vi "Powerstab.vi"(8 "error out":errorcluster, 10 "Power precision":dbl=0.1, 11 "Laser Power [W]":dbl format="%#.2g") -> (0 "error out 2":errorcluster, 3 "Finshed?":bool)   [LabVIEW 2011]
uses:
  monochromatorcontrol/perHandlemonochromator.vi
  GlobalVar.vi
  monochromatorcontrol/libPhyspec.lvlib
panel:
  out "error-1":dbl
  out "sum":dbl
  out "In Range?":bool
  out "Laser Q":dbl
  out "Laser Power":u8(slide) scale=0.0..2350.0
  out "Current Power":dbl
  out "Current Wavelength":dbl
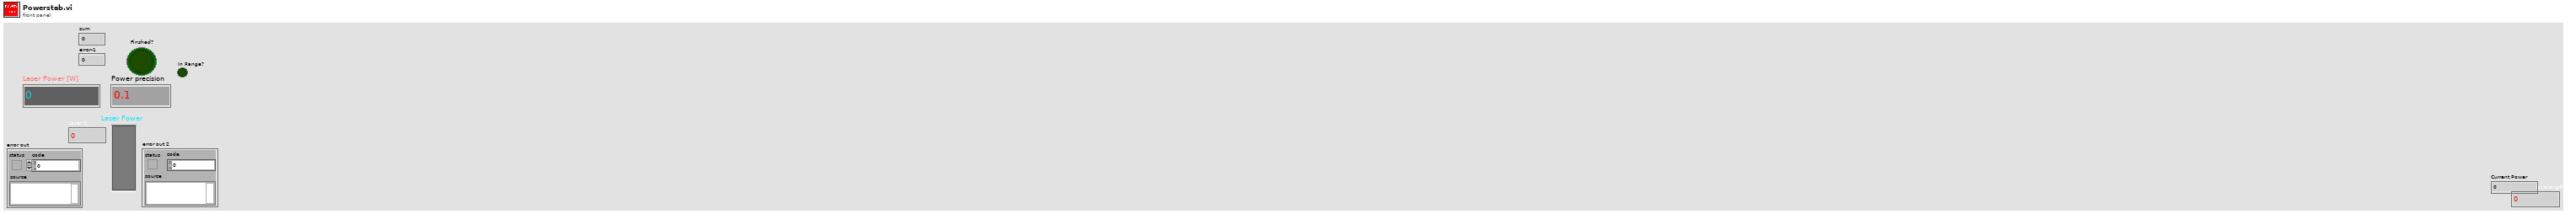
[diagram p1: front panel]
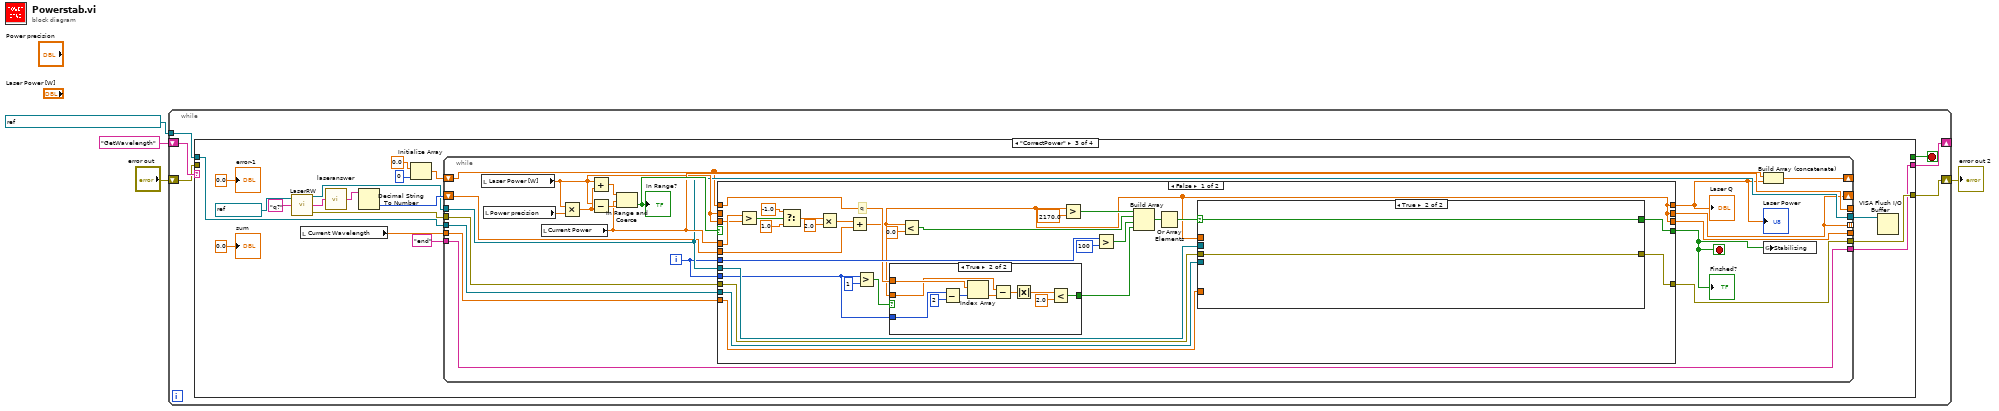
[diagram p0: block diagram]
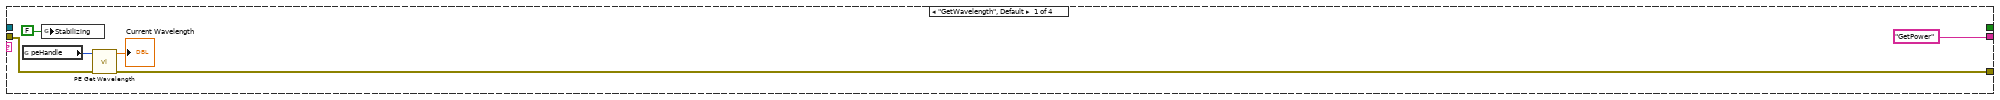
[diagram p2: hidden frame]
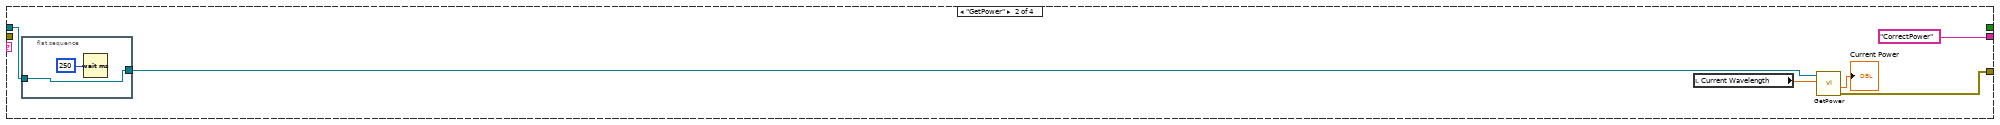
[diagram p3: hidden frame]
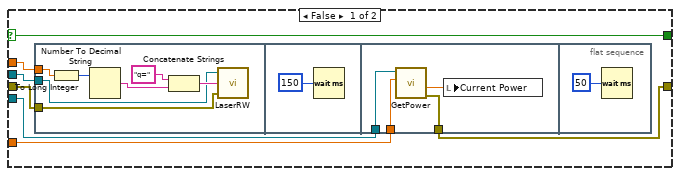
[diagram p5: hidden frame]
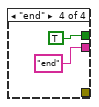
[diagram p7: hidden frame]
diagram:
  n1 = while {
    shift-right: [w7] -> _
    shift-left: "GetWavelength" -> [w10]
    shift-right: [w8] -> w1
    shift-left: "error out" -> [w9]
    tunnel: refnum<visa-resource-name> "USB0::0x1313::0x8072::P2007928::INSTR" ("Input Device") -> [w6]
    stop <- w5 stop-if-true
    n2 = case shown="\"CorrectPower\"" w10 {
      tunnel: w9 -> [w14 _ _ _]
      tunnel: [w13 w18 w27 _] -> w8
      tunnel: ["GetPower" "CorrectPower" w25 "end"] -> w7
      tunnel: w6 -> [_ w20 w29 _]
      tunnel: [_ _ _ TRUE] -> w5
      frame "GetWavelength", Default {
        n3 = global read "perHandlemonochromator.vi" "peHandle"() -> (w16:u32)
        n4 = global write "GlobalVar.vi" "Stabilizing"(FALSE ("Stabilizing")) -> ()
        n5 = call "PE Get Wavelength.vi"("error in (no error)"=w14, "peHandle"=w16) -> ("error out"=w13:errorcluster, "wavelength"=→"Current Wavelength":dbl)  [unwired: 7 in, 1 out]
      }
      frame "GetPower" {
        n6 = flat-sequence {
          tunnel: [w23] -> w21
          tunnel: w20 -> [w23]
          frame #0 {
            n7 = Wait (ms)(milliseconds to wait=u32 250) -> ()  [unwired: 1 out]
          }
        }
        n8 = local read "Current Wavelength"() -> (w19:dbl)
        n9 = call "GetPower.vi"("Wavelength (nm)"=w19, "Input Device"=w21) -> ("error out"=w18:errorcluster, "Power (W)"=→"Current Power":dbl)  [unwired: 2 in, 2 out]
      }
      frame "CorrectPower" {
        n10 = call "LaserRW.vi"("buffer à écrire"="q?", "Nom de ressource VISA"=refnum<visa-resource-name> "COM19") -> ("error out"=w36:errorcluster, "buffer lu"=w38:string, "Nom de ressource VISA en sortie"=w37:refnum<visa-resource-name>)  [unwired: 1 in]
        n11 = local read "Current Wavelength"() -> (w28:dbl)
        n12 = call "laseranswer.vi"("IN"=w38) -> ("Answer"=w35:string)
        n13 = Decimal String To Number(string=w35) -> (number=w39:i32)  [unwired: 2 in, 1 out]
        n14 = Initialize Array(0.0 ("element"), 0 ("dimension size")) -> (w31:dbl[])
        n15 = while {
          tunnel: [w58] -> _
          tunnel: w29 -> [w57]
          tunnel: w28 -> [w56]
          tunnel: [w55] -> _
          tunnel: w37 -> [w53]
          tunnel: [w53] -> w40
          shift-right: [w51] -> _
          shift-left: w39 -> [w50]
          tunnel: w36 -> [w52]
          tunnel: [w51] -> _ mode=indexing
          shift-right: [w48] -> _
          shift-left: w31 -> [w49]
          tunnel: [w45] -> w27
          tunnel: "end" -> [w44]
          tunnel: [w44] -> w25
          i -> [w47]
          stop <- w43 stop-if-true
          n16 = local read "Laser Power [W]"() -> (w54:dbl)
          n17 = local read "Power precision"() -> (w63:dbl)
          n18 = local read "Current Power"() -> (w58:dbl)
          n19 = Multiply(x=w54, y=w63) -> (x*y=w60:dbl)
          n20 = Add(x=w54, y=w60) -> (x+y=w61:dbl)
          n21 = Subtract(x=w54, y=w60) -> (x-y=w62:dbl)
          n22 = In Range and Coerce(upper limit=w61, x=w58, lower limit=w62) -> (In Range?=w59:bool)  [unwired: 1 out]
          "In Range?" <- w59
          n23 = case shown="False" w59 {
            selector: w59 -> [_ w129]
            tunnel: [w87 w129] -> w43
            tunnel: w58 -> [w86 _]
            tunnel: w54 -> [_ _]
            tunnel: w57 -> [w91 _]
            tunnel: w56 -> [w90 _]
            tunnel: w50 -> [w78 w128]
            tunnel: w53 -> [w92 _]
            tunnel: [w65 w128] -> w55
            tunnel: w47 -> [w71 _]
            tunnel: w54 -> [w85 _]
            tunnel: [w65 w128] -> w46
            tunnel: [w65 w128] -> w51
            tunnel: w52 -> [w77 w127]
            tunnel: w49 -> [w70 _]
            tunnel: w47 -> [w67 _]
            tunnel: [w64 w127] -> w45
            frame False {
              # "q"
              n24 = Greater?(x=w86, y=w85) -> (0:w84:bool)
              n25 = Select(t=-1.0, s=w84, f=1.0) -> (s? t:f=w81:dbl)
              n26 = Multiply(x=w81, y=2.0) -> (x*y=w79:dbl)
              n27 = Add(x=w79, y=w78) -> (x+y=w65:dbl)
              n28 = Greater?(x=w67, y=1) -> (0:w68:bool)
              n29 = case shown="True" w68 {
                selector: w68 -> [w94 _]
                tunnel: w70 -> [_ w103]
                tunnel: w67 -> [_ w102]
                tunnel: [w94 w95] -> w66
                tunnel: w65 -> [_ w101]
                frame False {
                }
                frame True {
                  n30 = Subtract(x=w102, y=2) -> (x-y=w104:i32)
                  n31 = Index Array(array=w103, index=w104) -> (element=w100:dbl)
                  n32 = Subtract(x=w101, y=w100) -> (x-y=w99:dbl)
                  n33 = Absolute Value(x=w99) -> (abs(x)=w96:dbl)
                  n34 = Less?(x=w96, y=2.0) -> (x < y?=w95:bool)
                }
              }
              n35 = Less?(x=w65, y=0.0) -> (x < y?=w75:bool)
              n36 = Greater?(x=w65, y=2170.0) -> (0:w76:bool)
              n37 = Greater?(x=w71, y=u32 100) -> (0:w74:bool)
              n38 = Build Array(w76, w75, w74, w66) -> (w73:bool[])
              n39 = Or Array Elements(Boolean array=w73) -> (logical OR=w72:bool)
              n40 = case shown="True" w72 {
                selector: w72 -> [w108 w126]
                tunnel: w92 -> [w111 _]
                tunnel: w91 -> [w110 _]
                tunnel: w90 -> [w109 _]
                tunnel: [w108 w126] -> w87
                tunnel: w77 -> [w107 w125]
                tunnel: w65 -> [w106 _]
                tunnel: [w105 w125] -> w64
                frame False {
                  n41 = flat-sequence {
                    tunnel: w111 -> [w113]
                    tunnel: w107 -> [w112]
                    tunnel: w106 -> [w114]
                    tunnel: w110 -> [w123]
                    tunnel: w109 -> [w122]
                    tunnel: [w120] -> w105
                    frame #0 {
                      n42 = To Long Integer(number=w114) -> (32bit integer=w117:i32)
                      n43 = Number To Decimal String(number=w117) -> (decimal integer string=w116:string)  [unwired: 1 in]
                      n44 = Concatenate Strings("q=" ("buffer à écrire"), w116) -> (w115:string)
                      n45 = call "LaserRW.vi"("error in (no error)"=w112, "buffer à écrire"=w115, "Nom de ressource VISA"=w113) -> ()  [unwired: 3 out]
                    }
                    frame #1 {
                      n46 = Wait (ms)(milliseconds to wait=u32 150) -> ()  [unwired: 1 out]
                    }
                    frame #2 {
                      n47 = call "GetPower.vi"("Wavelength (nm)"=w122, "Input Device"=w123) -> ("error out"=w120:errorcluster, "Power (W)"=w121:dbl)  [unwired: 2 in, 2 out]
                      n48 = local write "Current Power"(w121) -> ()
                    }
                    frame #3 {
                      n49 = Wait (ms)(milliseconds to wait=u32 50) -> ()  [unwired: 1 out]
                    }
                  }
                }
                frame True {
                }
              }
            }
            frame True {
            }
          }
          "Laser Q" <- w46
          "Laser Power" <- w46
          "Finshed?" <- w43
          n50 = Build Array (concatenate)(w49, w46) -> (w48:dbl[])
          n51 = global write "GlobalVar.vi" "Stabilizing"(w43) -> ()
        }
        n52 = VISA Flush I/O Buffer(VISA resource name=w40) -> ()  [unwired: 2 in, 2 out]
        "sum" <- 0.0
        "error-1" <- 0.0 ("differential")
      }
      frame "end" {
      }
    }
  }
  "error out 2" <- w1
